vi "Handle SREF XY.vi"(8 "error in":errorcluster, 11 "Referential in":refnum<class "Referential.lvclass">) -> (0 "error out":errorcluster, 2 "Transformation":cluster{"XY Matrix":T1}[](array[cluster]), 3 "Referential out":refnum<class "Referential.lvclass">)   [LabVIEW 2019, in "Referential.lvclass"]
uses:
  Referential.lvclass
  <vilib>/Analysis/Matrix/Datatypes/RealMatrix.ctl
  <vilib>/Analysis/baseanly.llb/Real A x B.vi
  <vilib>/Analysis/NI_AALBase.lvlib
  <vilib>/Analysis/Matrix/NI_Matrix.lvlib
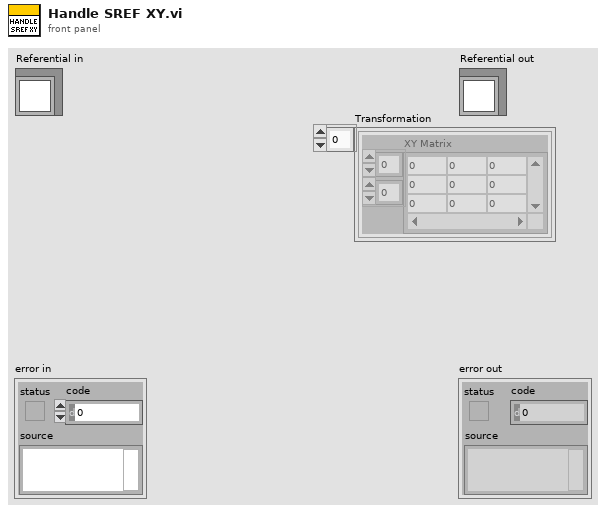
[diagram p1: front panel]
types:
  T1 = typedef "NI_Matrix.lvlib/RealMatrix.ctl" = dbl[][]
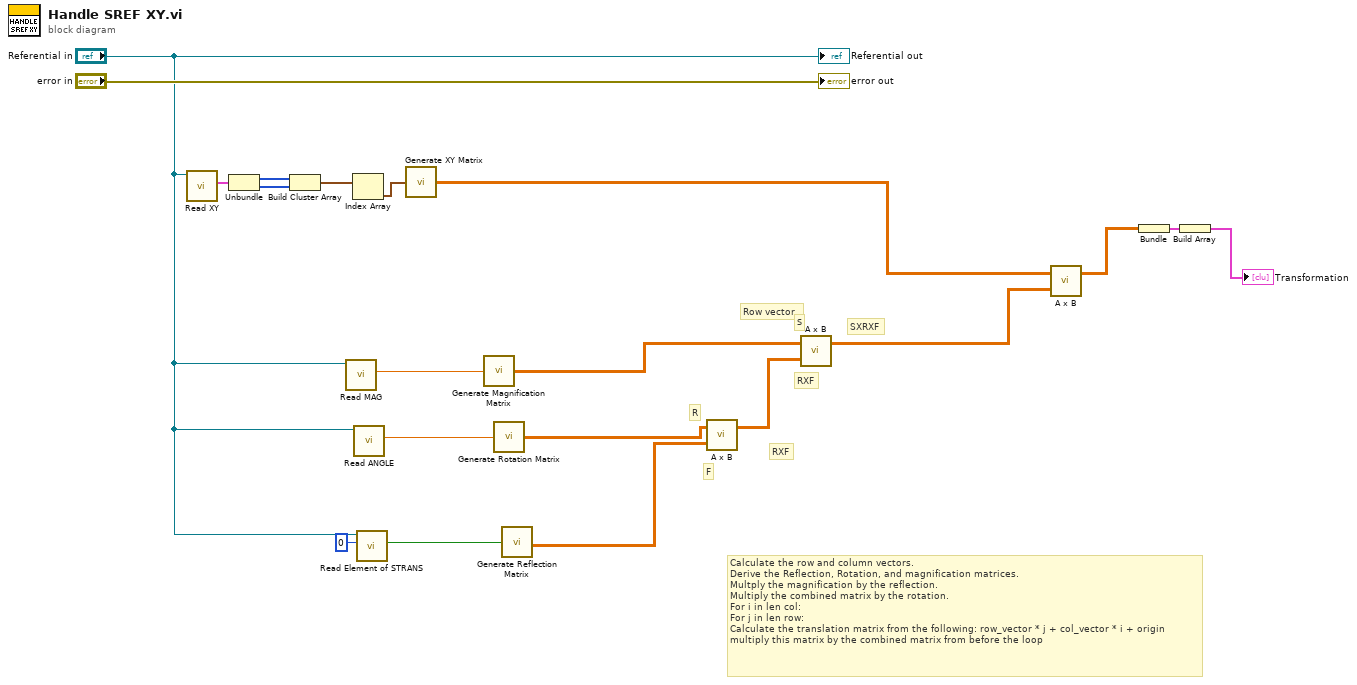
[diagram p0: block diagram]
diagram:
  # "SXRXF"
  # "RXF"
  # "S"
  # "RXF"
  # "R"
  # "F"
  # "Calculate the row and column vectors.\nDerive the Reflection, Rotation, and magnification matrices. \nMultply the magnification by the reflection.\nMultiply the combined matrix by the rotation.\nFor i in len col:\nFor j in len row:\nCalculate the translation matrix from the following: row_vector * j + col_vector * i + origin\nmultiply this matrix by the combined matrix from before the loop"
  # "Row vector"
  n1 = call-dynamic "Read XY.vi"("Element in"="Referential in") -> ("XY"=w18:cluster{"X":i32[], "Y":i32[]})  [unwired: 8 in, 2 out]
  n2 = Unbundle(w18) -> ("X"=w16:i32[], "Y"=w15:i32[])
  n3 = Build Cluster Array(w16, w15) -> (w14:cluster{"X":i32, "X":i32}[])
  n4 = call-dynamic "Read MAG.vi"("Referential in"="Referential in") -> ("MAG"=w8:dbl)  [unwired: 8 in, 2 out]
  n5 = Index Array(array=w14) -> (element=w17:cluster{"X":i32, "X":i32})  [unwired: 1 in]
  n6 = call-dynamic "Read ANGLE.vi"("Referential in"="Referential in") -> ("ANGLE"=w9:dbl)  [unwired: 8 in, 2 out]
  n7 = call-dynamic "Read Element of STRANS.vi"("index"=0, "Referential in"="Referential in") -> ("Bit"=w3:bool)  [unwired: 7 in, 2 out]
  n8 = call "Generate XY Matrix.vi"("XY"=w17) -> ("XY Matrix"=w11:T1)
  n9 = call "Generate Magnification Matrix.vi"("Magnification"=w8) -> ("Magnification Matrix"=w7:T1)
  n10 = call "Generate Rotation Matrix.vi"("Angle"=w9) -> ("Rotation Matrix"=w6:T1)
  n11 = call "Generate Reflection Matrix.vi"("Bit"=w3) -> ("Reflection Matrix"=w4:T1)
  n12 = call-poly <vilib>:"A x B.vi"("B"=w4, "A"=w6) -> ("A x B"=w5:T1)  [unwired: 1 out]
  n13 = call-poly <vilib>:"A x B.vi"("B"=w5, "A"=w7) -> ("A x B"=w2:T1)  [unwired: 1 out]
  n14 = call-poly <vilib>:"A x B.vi"("B"=w2, "A"=w11) -> ("A x B"=w13:T1)  [unwired: 1 out]
  n15 = Bundle("A x B"=w13) -> (w19:cluster{"A x B":T1})  [unwired: 1 in]
  n16 = Build Array(w19) -> (→"Transformation":cluster{"A x B":T1}[])
  "error out" <- "error in"
  "Referential out" <- "Referential in"
